vi "main.vi"() -> ()   [LabVIEW 2021, in "material--ppl--target.lvlib"]
uses:
  material--ppl--target.lvlib
panel:
  in  "File Path (theme)":path
  in  "filled--text--rectangular":bool
  in  "tonal--icons--rounded":bool
  in  "outline--text--rectangular":bool
  in  "FAB Button":bool
  # "control UI role = Primary"
  # "control UI role = Primary"
  # "Decoration--Surface Container Low"
  # "control UI role = Tertiary"
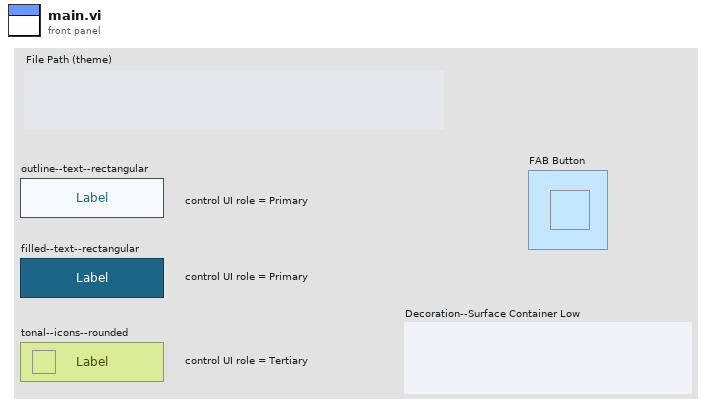
[diagram p1: front panel]
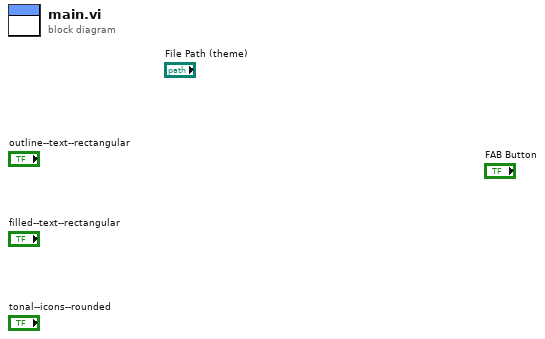
[diagram p0: block diagram]
diagram:
